vi "Gserver_main.vi"(8 "Database location":path=path "D:/Sgraph_database", 11 "DAQ-Queue":refnum<queue>) -> ()   [LabVIEW 2020, in "Gserver.lvclass"]
doc: "Gserver service.\n\nThis service will act on Gviewer queries.\nThis VI must be started to enable the Sgraph functionality\n\nUse the Close method of the Gserver class after the main application is ended to free all resources."
uses:
  Gserver.lvclass
  controls/Typedef_Gserver-init.ctl
  HISW/controls/typedef-DAQ-datagram.ctl
  HISW/controls/typedef-Qtype.ctl
  Gview/controls/Typedef_datarequest.ctl
  Gview/controls/Typedef_Live.ctl
  FAMM/controls/FAMM_reply_datagram.ctl
  FAMM/controls/FAMM_reply_WAQdata.ctl
  FAMM/controls/FAMM_reply_EAQdata.ctl
  FAMM/controls/FAMM_reply_PAQdata.ctl
  D:/Labview/Sgraph/Sgraph/source/Vsolver/Vsolver.lvclass
  Gserver.lvclass/Gserver.ctl
  Common/controls/MeMapInfo.ctl
  Common/controls/MMap_element.ctl
  FAMM/controls/typedef-functions.ctl
  controls/Typedef_Sgraph_Query.ctl
  Gview/controls/Typedef_Gserver-Replies.ctl
  Gview/controls/Typedef_ServerActions.ctl
  FAMM/FAMM.lvclass/FAMM.ctl
  FAMM/FAMM.lvclass
  HISW/HISW.lvclass
  FAMM/controls/typedef_FAMM_Query.ctl
  Common/controls/Global-services.vi
  Vsolver/Vsolver.lvclass
  Gview/Gviewer.lvclass
panel:
  out "Debug_Layer?":i32
  out "data 2":T1
  out "data":T6
  out "# elements in queue":i32
  out "Graphs Running":string[](array[string])
  out "Gserver":picture
  out "GserverInitState":T7
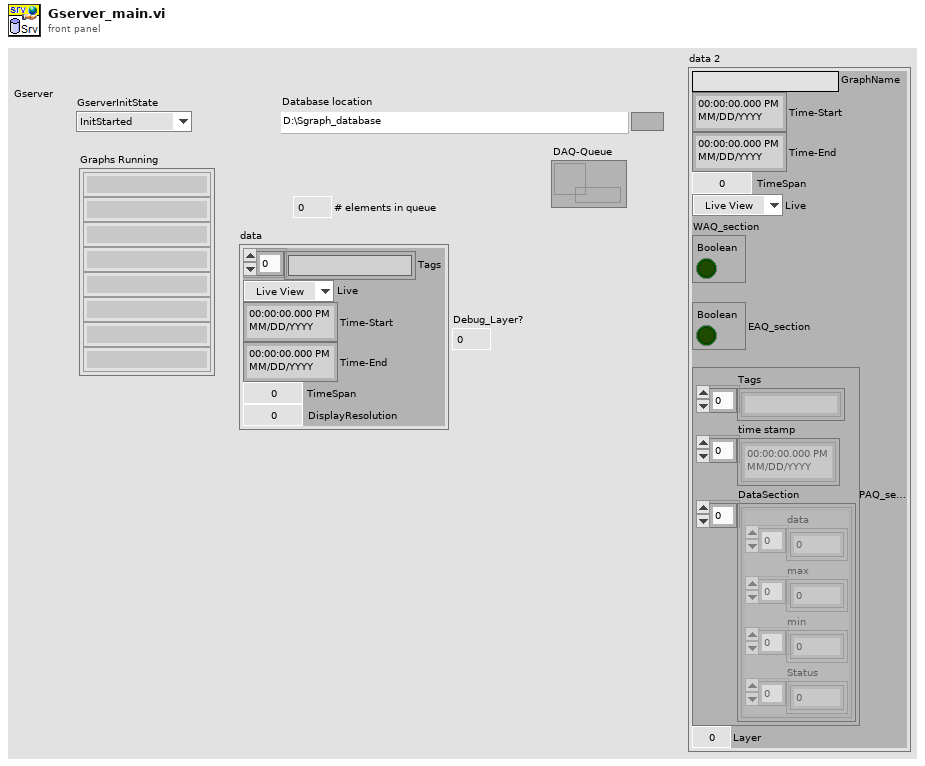
[diagram p1: front panel]
types:
  T1 = typedef "FAMM.lvclass/FAMM_reply_datagram.ctl" = cluster{"GraphName":string, "Time-Start":timestamp, "Time-End":timestamp, "TimeSpan":dbl, "Live":T2, "WAQ_section":T3, "EAQ_section":T4, "PAQ_section":T5, "Layer":i32}
  T2 = typedef "Gviewer.lvclass/Typedef_Live.ctl" = enum16{"Live View", "Freeze"}
  T3 = typedef "FAMM.lvclass/FAMM_reply_WAQdata.ctl" = cluster{"Boolean":bool}
  T4 = typedef "FAMM.lvclass/FAMM_reply_EAQdata.ctl" = cluster{"Boolean":bool}
  T5 = typedef "FAMM.lvclass/FAMM_reply_PAQdata.ctl" = cluster{"Tags":string[], "time stamp":timestamp[], "DataSection":cluster{"data":dbl[], "max":dbl[], "min":dbl[], "Status":u32[]}[]}
  T6 = typedef "Gviewer.lvclass/Typedef_datarequest.ctl" = cluster{"Tags":string[], "Live":T2, "Time-Start":timestamp, "Time-End":timestamp, "TimeSpan":dbl, "DisplayResolution":i32}
  T7 = typedef "Typedef_Gserver-init.ctl" = enum16{"InitStarted", "FAMM_started", "HISW_Started", "Active"}
  T8 = typedef "typedef-functions.ctl" = enum16{"PAQ-request", "PAQ-taglist-request", "WAQ-request", "EAQ-request", "TAG-based-request", "PAQ-MemoryMap", "Exit-FAMM"}
  T9 = typedef "MeMapInfo.ctl" = cluster{"MemLayer":T10[]}
  T10 = typedef "MMap_element.ctl" = cluster{"Name":string, "Length":i32, "Pointer":i32, "Tbegin":dbl, "Tend":dbl, "Tmin":dbl, "Tmax":dbl, "Tpnt-1":dbl, "Tpnt":dbl, "Tpnt+1":dbl}
  T11 = typedef "Gserver.lvclass/Typedef_Sgraph_Query.ctl" = cluster{"ViewportName":string, "Tags":string[], "Time-Start":timestamp, "Time-End":timestamp, "Pixels":i32, "Live":T2, "TimeSpan(sec)":dbl, "GViewer-Queue":refnum<queue>}
  T12 = typedef "Typedef_ServerActions.ctl" = enum16{"GraphUpdate", "SendAllTags", "SendIniPath", "SetGeneralOptions", "EditTagsOpen", "EditTagsPresetSave", "EditTagsPresetLoad", "EditTagsClose", "NewTagSelection", "ExitGraph"}
  T13 = typedef "Typedef_Gserver-Replies.ctl" = cluster{"ServerActions":T12, "data":variant, "Source":string, "Time Stamp":timestamp}
  T14 = typedef "typedef-Qtype.ctl" = enum16{"PAQ", "WAQ", "EAQ", "End-Service"}
  T15 = typedef "typedef-DAQ-datagram.ctl" = cluster{"Time Stamp":timestamp, "Source":string, "Data":variant, "Qtype":T14}
  T16 = typedef "typedef_FAMM_Query.ctl" = cluster{"Time Stamp":timestamp, "FAMM-function":T8, "Source":string, "Data":variant}
  T17 = typedef "Gserver.lvclass/Typedef_Gviewer-Query.ctl" = cluster{"Query_type":T18, "data":variant, "Source":string, "Time Stamp":timestamp}
  T18 = typedef "Gserver.lvclass/Typedef_QueryType.ctl" = enum16{"Subscribe", "DataRequest", "RequestAllTags", "RequestIniPath", "FAMMstarted", "SetClientOptions", "GviewerUpdate", "OpenNewGraph", "CloseClient", "CloseAllClients", "Close Gserver", "OpenMemoryMap", "MeMapDataRequest", "MeMapDataResponse"}
  T19 = typedef "FAMM.lvclass/Typedef_Gviewer_TagsUnits.ctl" = cluster{"PAQ_TAGs":string[], "WAQ_TAGs":string[], "EAQ_TAGs":string[], "PAQtagProps":T20[], "WAQtagProps":T20[], "EAQtagProps":T20[]}
  T20 = typedef "typedef_com_TagProp.ctl" = cluster{"Description":string, "EngUnits":string, "RangeH":dbl, "RangeL":dbl, "Resolution":i32, "Obsolete":bool, "ChangeDate":timestamp, "ChangeSource":string, "ChangeReason":string, "TagFunc":u32}
  T21 = cluster{"FAMM_PAQ_Layers":i32, "FAMM_PAQ_resolution":dbl}
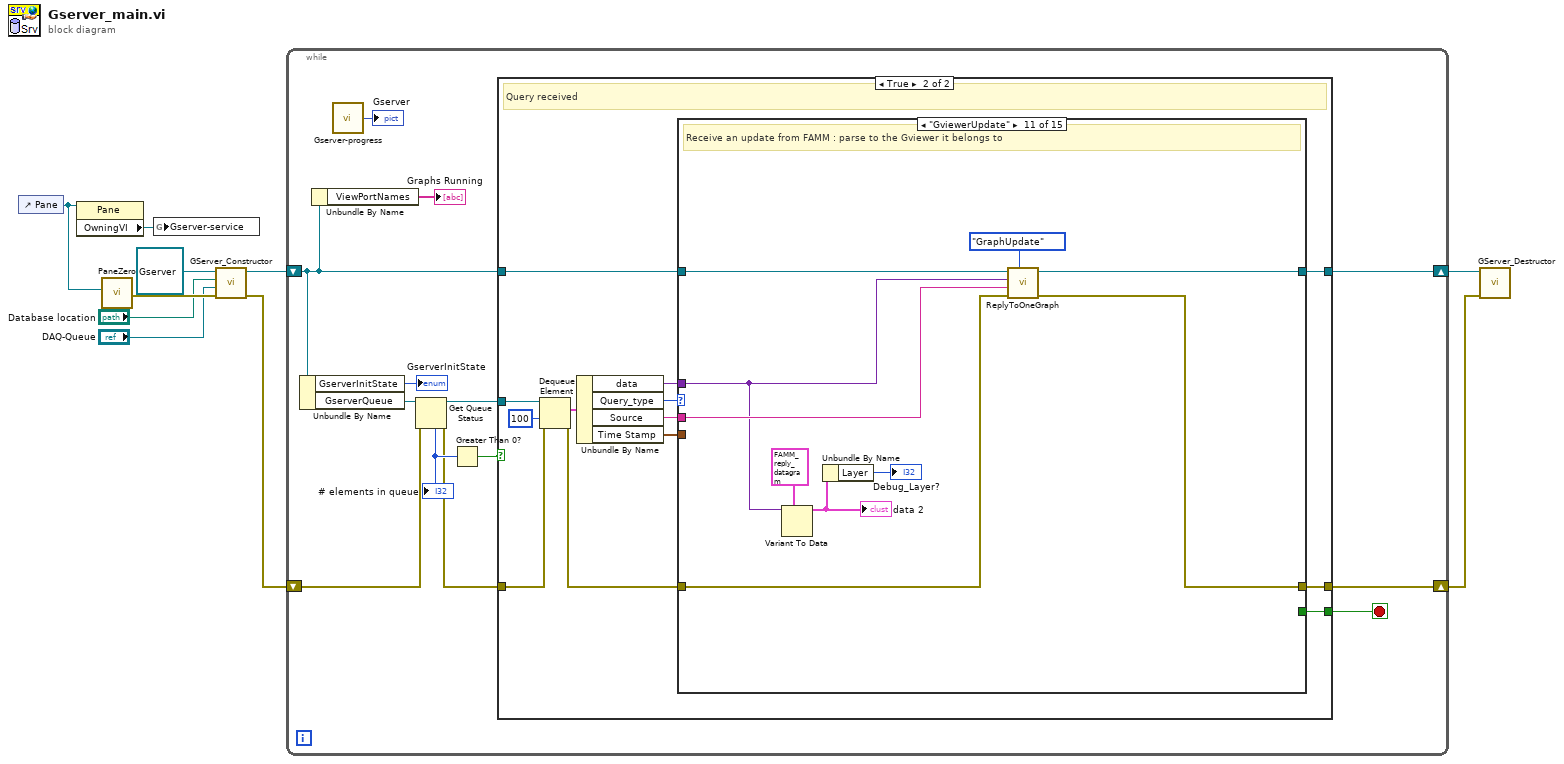
[diagram p0: block diagram]
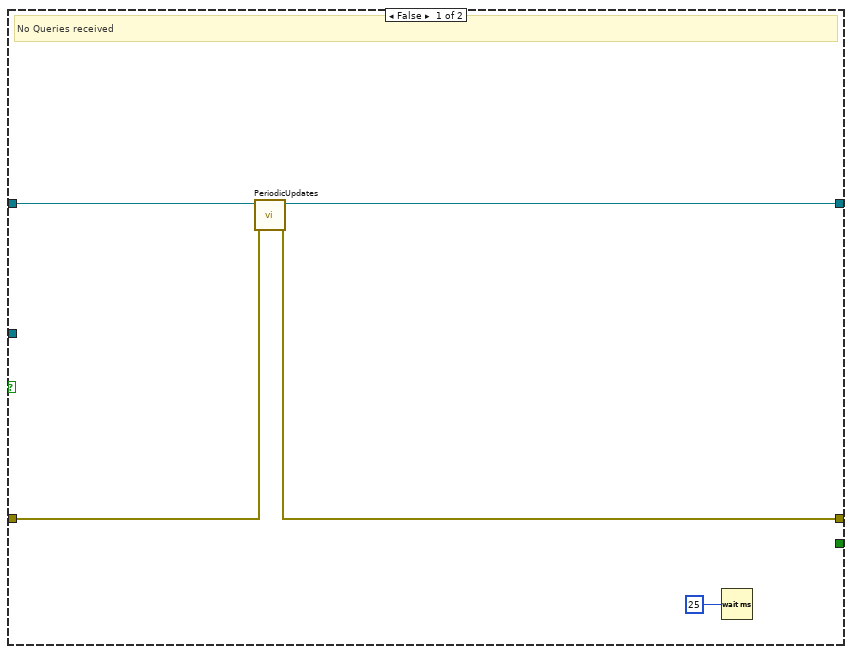
[diagram p2: hidden frame]
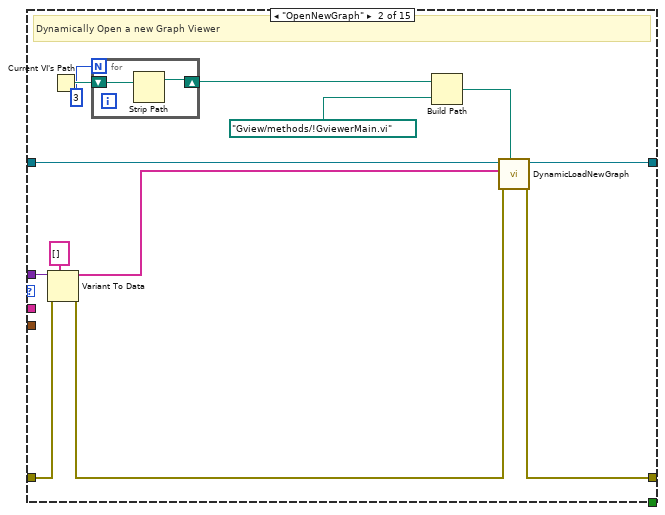
[diagram p4: hidden frame]
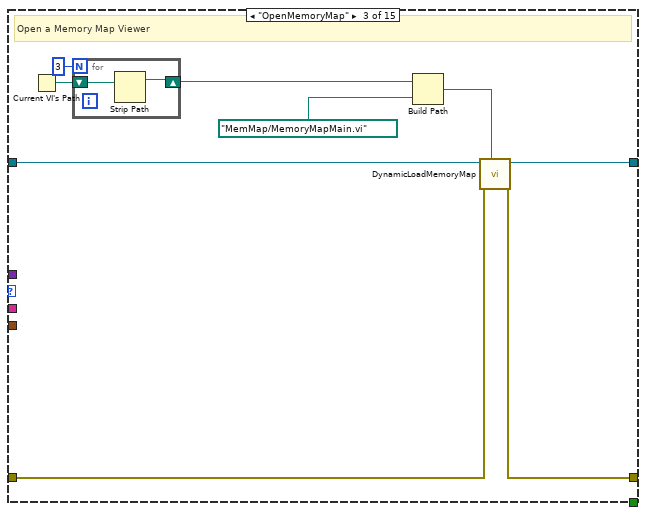
[diagram p5: hidden frame]
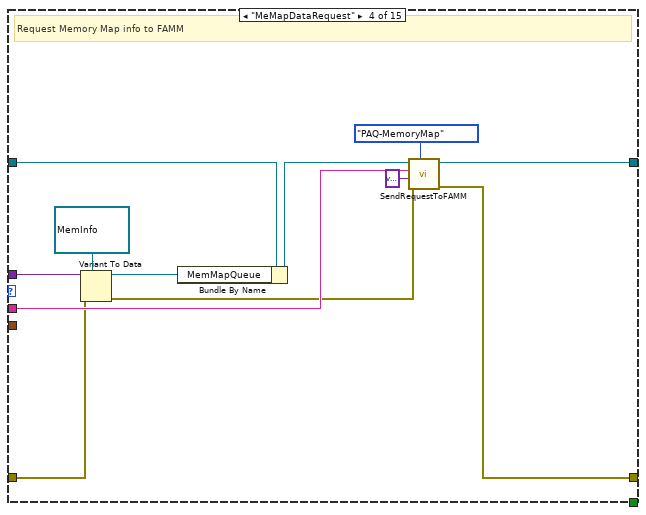
[diagram p6: hidden frame]
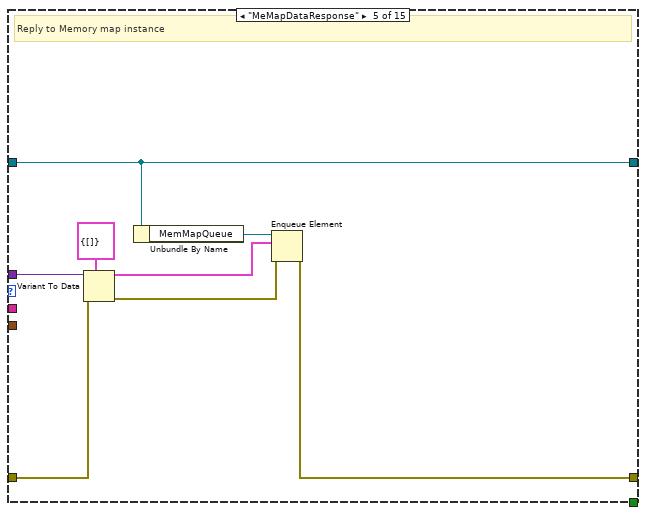
[diagram p7: hidden frame]
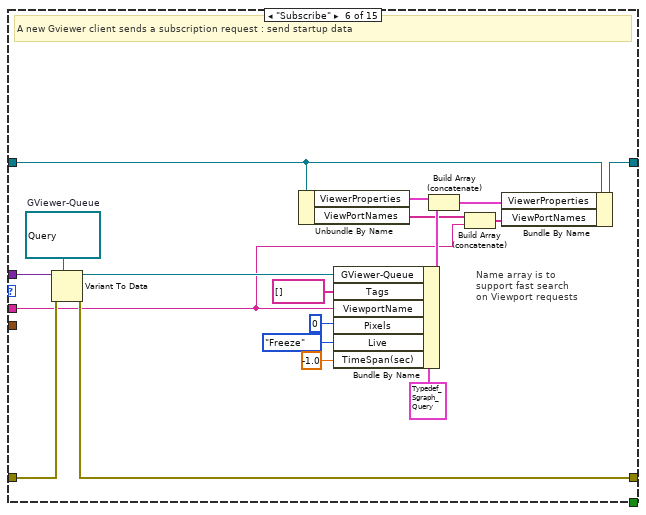
[diagram p8: hidden frame]
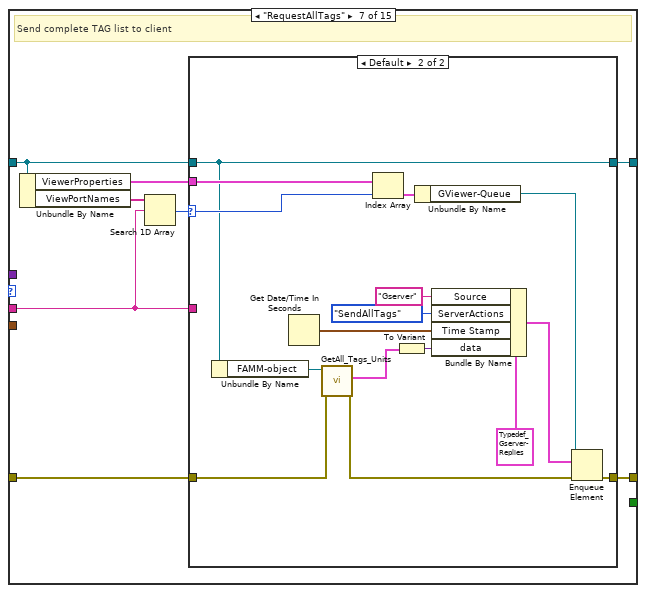
[diagram p9: hidden frame]
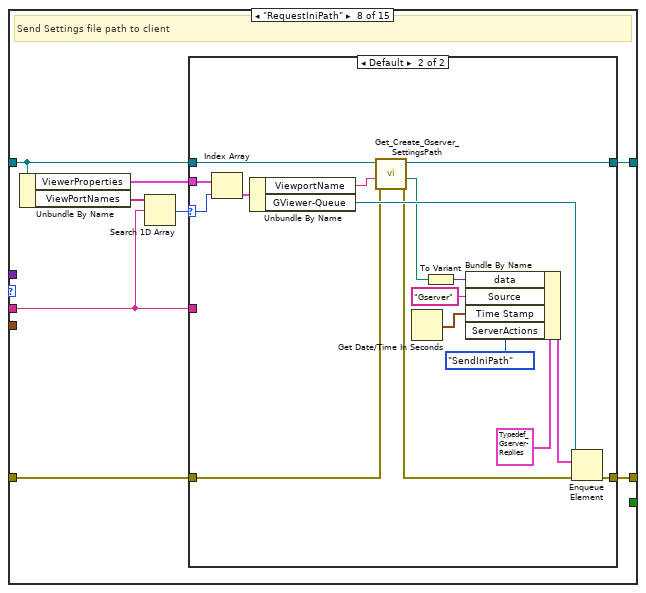
[diagram p11: hidden frame]
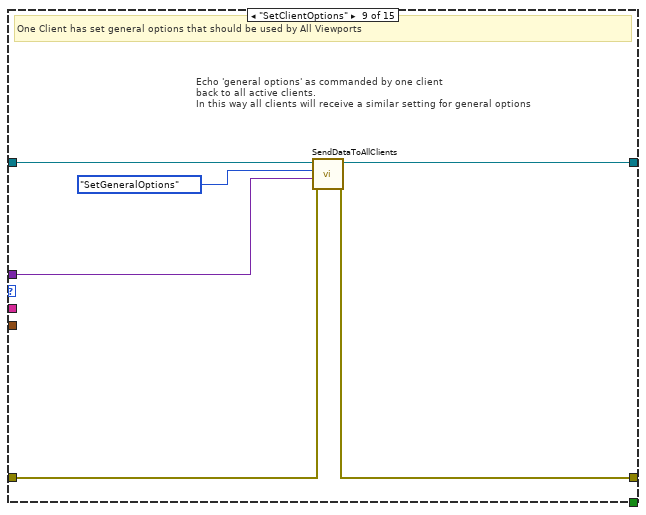
[diagram p13: hidden frame]
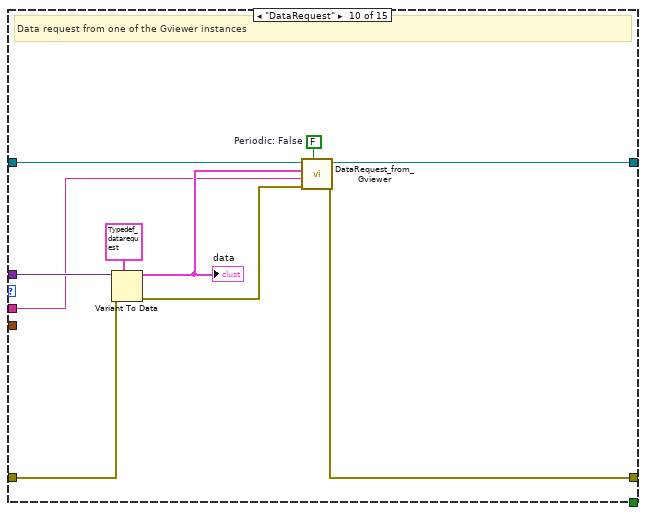
[diagram p14: hidden frame]
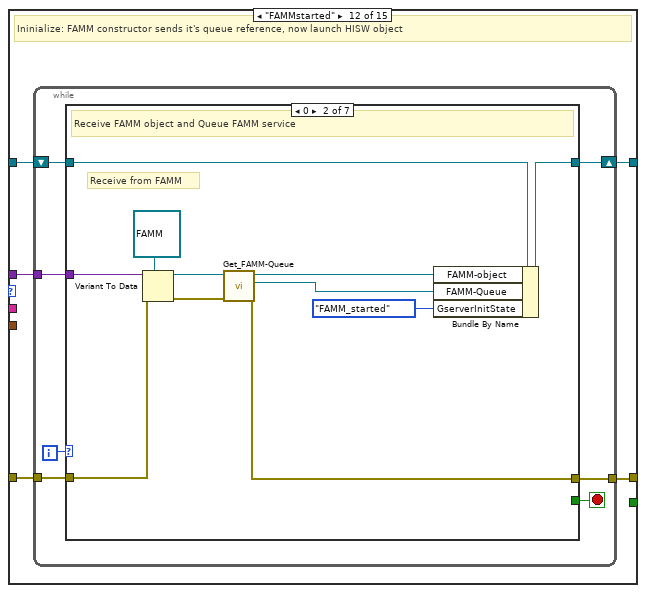
[diagram p15: hidden frame]
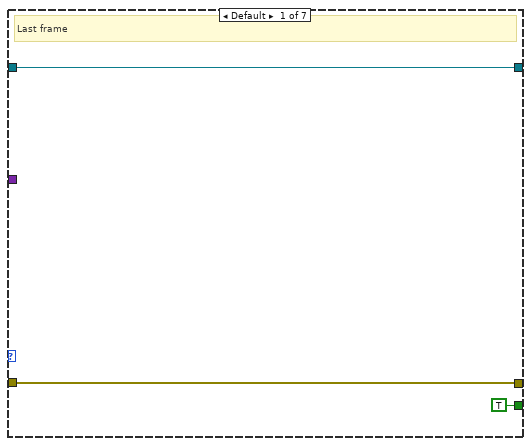
[diagram p16: hidden frame]
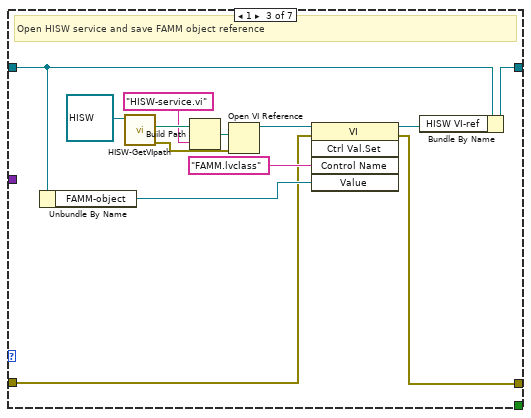
[diagram p17: hidden frame]
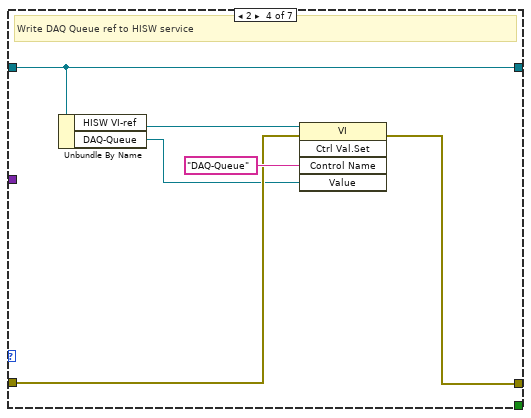
[diagram p18: hidden frame]
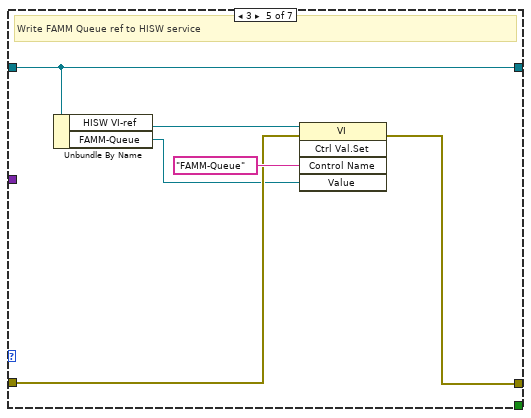
[diagram p19: hidden frame]
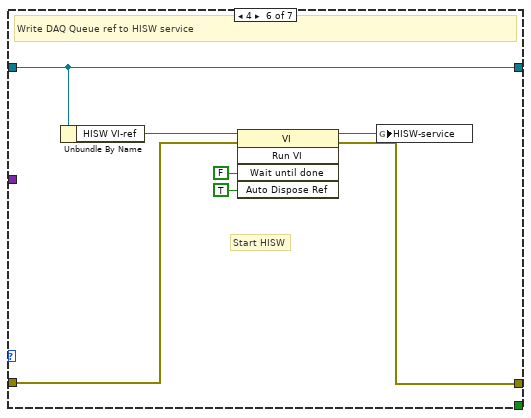
[diagram p20: hidden frame]
diagram:
  n1 = control-ref of="Pane"() -> (w3:refnum<vi>)
  n2 = property class="Pane"(reference=w3) -> ("OwningVI"=w5:refnum<vi>)  [unwired: 1 in, 2 out]
  n3 = call "PaneZero.vi"("Pane"=w3) -> ("error out"=w4:errorcluster)  [unwired: 10 in]
  n4 = global write "Global-services.vi" "Gserver-service"(w5) -> ()
  n5 = call "GServer_Constructor.vi"("error in (no error)"=w4, "DAQ-Queue"="DAQ-Queue", "Database location"="Database location", "Gserver in"=refnum<class "Gserver.lvclass"> refnum) -> ("error out"=w9:errorcluster, "Gserver out"=w10:refnum<class "Gserver.lvclass">)  [unwired: 6 in]
  n6 = while {
    shift-right: [w20] -> w8
    shift-left: w10 -> [w12]
    shift-right: [w19] -> w7
    shift-left: w9 -> [w17]
    stop <- w13 stop-if-true
    n7 = Unbundle By Name(w12) -> ("GserverInitState"=→"GserverInitState":T7, "GserverQueue"=w23:refnum<queue>)
    n8 = Unbundle By Name(w12) -> ("ViewPortNames"=→"Graphs Running":string[])
    n9 = call "Gserver-progress.vi"() -> ("37x37"=→"Gserver":picture)  [unwired: 7 in]
    n10 = Get Queue Status(queue=w23, error in (no error)=w17) -> (queue out=w18:refnum<queue>, error out=w16:errorcluster, # elements in queue=w22:i32)  [unwired: 1 in, 5 out]
    "# elements in queue" <- w22
    n11 = Greater Than 0?(x=w22) -> (x > 0?=w21:bool)
    n12 = case shown="True" w21 {
      tunnel: w12 -> [w27 w35]
      tunnel: w16 -> [w26 w39]
      tunnel: [w25 w33] -> w20
      tunnel: [w24 w34] -> w19
      tunnel: w18 -> [_ w41]
      tunnel: [_ w30] -> w13
      frame False {
        # "No Queries received"
        n13 = call "PeriodicUpdates.vi"("error in (no error)"=w26, "Gserver in"=w27) -> ("error out"=w24:errorcluster, "Gserver out"=w25:refnum<class "Gserver.lvclass">)  [unwired: 8 in]
        n14 = Wait (ms)(milliseconds to wait=u32 25) -> ()  [unwired: 1 out]
      }
      frame True {
        # "Query received"
        n15 = Dequeue Element(queue=w41, timeout in ms (-1)=100, error in (no error)=w39) -> (element=w38:T17, error out=w36:errorcluster)  [unwired: 2 out]
        n16 = Unbundle By Name(w38) -> ("data"=w32:variant, "Query_type"=w37:T18, "Source"=w29:string, "Time Stamp"=w31:timestamp)
        n17 = case shown="\"GviewerUpdate\"" w37 {
          tunnel: w36 -> [w42 w44 w60 w71 w82 w93 w111 w137 w162 w174 w182 w188 w255 w261 w272]
          tunnel: w35 -> [w43 w49 w62 w78 w89 w107 w113 w139 w166 w172 w186 w190 w257 w260 w271]
          tunnel: [w42 w48 w61 w72 w83 w94 w110 w136 w161 w168 w184 w187 w254 w258 w269] -> w34
          tunnel: [w43 w50 w63 w75 w89 w106 w112 w138 w165 w173 w185 w191 w256 w259 w270] -> w33
          tunnel: w32 -> [_ w56 _ w81 w87 w97 _ _ w163 w176 w179 w189 _ _ _]
          tunnel: w31 -> [_ _ _ _ _ _ _ _ _ _ _ _ _ _ _]
          tunnel: [_ _ _ _ _ _ _ _ _ _ _ _ _ _ w268] -> w30
          tunnel: w29 -> [_ _ _ w74 _ w90 w114 w140 _ w169 w183 _ w253 _ _]
          frame Default {
            # "Not implemented"
          }
          frame "OpenNewGraph" {
            # "Dynamically Open a new Graph Viewer"
            n18 = Variant To Data(error in=w44, type=string[] [], Variant=w56) -> (data=w46:string[], error out=w45:errorcluster)
            n19 = Current VI's Path() -> (path=w54:path)
            n20 = for {
              N: 3 -> [_]
              shift-right: [w57] -> w52
              shift-left: w54 -> [w58]
              n21 = Strip Path(path=w58) -> (stripped path=w57:path)  [unwired: 1 out]
            }
            n22 = Build Path(base path=w52, name or relative path=path "Gview/methods/!GviewerMain.vi") -> (appended path=w47:path)
            n23 = call "DynamicLoadNewGraph.vi"("ViewerPath"=w47, "error in (no error)"=w45, "Preferred_tags"=w46, "Gserver in"=w49) -> ("error out"=w48:errorcluster, "Gserver out"=w50:refnum<class "Gserver.lvclass">)  [unwired: 6 in]
          }
          frame "OpenMemoryMap" {
            # "Open a Memory Map Viewer"
            n24 = Current VI's Path() -> (path=w67:path)
            n25 = for {
              N: 3 -> [_]
              shift-right: [w68] -> w65
              shift-left: w67 -> [w69]
              n26 = Strip Path(path=w69) -> (stripped path=w68:path)  [unwired: 1 out]
            }
            n27 = Build Path(base path=w65, name or relative path=path "MemMap/MemoryMapMain.vi") -> (appended path=w59:path)
            n28 = call "DynamicLoadMemoryMap.vi"("ApplicationPath"=w59, "error in (no error)"=w60, "Gserver in"=w62) -> ("error out"=w61:errorcluster, "Gserver out"=w63:refnum<class "Gserver.lvclass">)  [unwired: 7 in]
          }
          frame "MeMapDataRequest" {
            # "Request Memory Map info to FAMM"
            n29 = Variant To Data(error in=w71, type=refnum<queue> refnum ("queue out"), Variant=w81) -> (data=w79:refnum<queue>, error out=w73:errorcluster)
            n30 = Bundle By Name(cluster=w78, "MemMapQueue"=w79) -> (w76:refnum<class "Gserver.lvclass">)
            n31 = call "SendRequestToFAMM.vi"("FAMM-function"=typedef-functions."PAQ-MemoryMap", "error in (no error)"=w73, "Data"=variant, "Source"=w74, "Gserver in"=w76) -> ("error out"=w72:errorcluster, "Gserver out"=w75:refnum<class "Gserver.lvclass">)  [unwired: 5 in]
          }
          frame "MeMapDataResponse" {
            # "Reply to Memory map instance"
            n32 = Variant To Data(error in=w82, type=T9 {"MemLayer"=[]} ("element"), Variant=w87) -> (data=w84:T9, error out=w85:errorcluster)
            n33 = Unbundle By Name(w89) -> ("MemMapQueue"=w88:refnum<queue>)
            n34 = Enqueue Element(queue=w88, element=w84, error in (no error)=w85) -> (error out=w83:errorcluster)  [unwired: 1 in, 2 out]
          }
          frame "Subscribe" {
            w98 = refnum<queue> refnum  # GViewer-Queue
            # "Name array is to\nsupport fast search\non Viewport requests"
            # "A new Gviewer client sends a subscription request : send startup data"
            n35 = Variant To Data(error in=w93, type=w98, Variant=w97) -> (data=w96:refnum<queue>, error out=w94:errorcluster)
            n36 = Unbundle By Name(w107) -> ("ViewerProperties"=w105:T11[], "ViewPortNames"=w92:string[])
            n37 = Bundle By Name(cluster=T11 {"ViewportName"="", "Tags"=[], "Time-Start"=timestamp(0 s since 1904-01-01), "Time-End"=timestamp(0 s since 1904-01-01), "Pixels"=0, "Live"=enum."Live View", "TimeSpan(sec)"=0.0, "GViewer-Queue"=refnum} ("Query_datagram"), "GViewer-Queue"=w96, "Tags"=string[] [], "ViewportName"=w90, "Pixels"=0, "Live"=Typedef_Live."Freeze", "TimeSpan(sec)"=-1.0) -> (w102:T11)
            n38 = Build Array (concatenate)(w105, w102) -> (w104:T11[])
            n39 = Build Array (concatenate)(w92, w90) -> (w91:string[])
            n40 = Bundle By Name(cluster=w107, "ViewerProperties"=w104, "ViewPortNames"=w91) -> (w106:refnum<class "Gserver.lvclass">)
          }
          frame "RequestAllTags" {
            # "Send complete TAG list to client"
            n41 = Unbundle By Name(w113) -> ("ViewerProperties"=w109:T11[], "ViewPortNames"=w115:string[])
            n42 = Search 1D Array(1D array=w115, element=w114) -> (index of element=w108:i32)  [unwired: 1 in]
            n43 = case shown="Default" w108 {
              selector: w108 -> [_ w132]
              tunnel: w114 -> [_ _]
              tunnel: w113 -> [w117 w128]
              tunnel: [w117 w128] -> w112
              tunnel: w111 -> [w116 w120]
              tunnel: [w116 w129] -> w110
              tunnel: w109 -> [_ w133]
              frame -1 {
              }
              frame Default {
                n44 = Unbundle By Name(w128) -> ("FAMM-object"=w121:refnum<class "FAMM.lvclass">)
                n45 = Get Date/Time In Seconds() -> (seconds since 1Jan1904=w124:timestamp)
                n46 = call "GetAll_Tags_Units.vi"("error in (no error)"=w120, "FAMM in"=w121) -> ("error out"=w119:errorcluster, "Tags_Units"=w118:T19)  [unwired: 7 in, 1 out]
                n47 = Index Array(array=w133, index=w132) -> (element=w131:T11)
                n48 = To Variant(anything=w118) -> (Variant=w122:variant)
                n49 = Unbundle By Name(w131) -> ("GViewer-Queue"=w130:refnum<queue>)
                n50 = Bundle By Name(cluster=T13 {"ServerActions"=enum."GraphUpdate", "data"=variant, "Source"="", "Time Stamp"=timestamp(0 s since 1904-01-01)} ("element"), "Source"="Gserver", "ServerActions"=Typedef_ServerActions."SendAllTags", "Time Stamp"=w124, "data"=w122) -> (w126:T13)
                n51 = Enqueue Element(queue=w130, element=w126, error in (no error)=w119) -> (error out=w129:errorcluster)  [unwired: 1 in, 2 out]
              }
            }
          }
          frame "RequestIniPath" {
            # "Send Settings file path to client"
            n52 = Unbundle By Name(w139) -> ("ViewerProperties"=w135:T11[], "ViewPortNames"=w141:string[])
            n53 = Search 1D Array(1D array=w141, element=w140) -> (index of element=w134:i32)  [unwired: 1 in]
            n54 = case shown="Default" w134 {
              selector: w134 -> [_ w159]
              tunnel: w140 -> [_ _]
              tunnel: w139 -> [w143 w151]
              tunnel: [w143 w152] -> w138
              tunnel: w137 -> [w142 w148]
              tunnel: [w142 w156] -> w136
              tunnel: w135 -> [_ w160]
              frame -1 {
              }
              frame Default {
                n55 = Index Array(array=w160, index=w159) -> (element=w158:T11)
                n56 = Unbundle By Name(w158) -> ("ViewportName"=w150:string, "GViewer-Queue"=w157:refnum<queue>)
                n57 = call "Get_Create_Gserver_SettingsPath.vi"("error in (no error)"=w148, "ViewPortName"=w150, "Gserver in"=w151) -> ("error out"=w149:errorcluster, "Viewport settings path"=w144:path, "Gserver out"=w152:refnum<class "Gserver.lvclass">)  [unwired: 6 in]
                n58 = Get Date/Time In Seconds() -> (seconds since 1Jan1904=w146:timestamp)
                n59 = To Variant(anything=w144) -> (Variant=w147:variant)
                n60 = Bundle By Name(cluster=T13 {"ServerActions"=enum."GraphUpdate", "data"=variant, "Source"="", "Time Stamp"=timestamp(0 s since 1904-01-01)} ("element"), "data"=w147, "Source"="Gserver", "Time Stamp"=w146, "ServerActions"=Typedef_ServerActions."SendIniPath") -> (w154:T13)
                n61 = Enqueue Element(queue=w157, element=w154, error in (no error)=w149) -> (error out=w156:errorcluster)  [unwired: 1 in, 2 out]
              }
            }
          }
          frame "SetClientOptions" {
            # "Echo 'general options' as commanded by one client\nback to all active clients.\nIn this way all clients will receive a similar setting for general options"
            # "One Client has set general options that should be used by All Viewports"
            n62 = call "SendDataToAllClients.vi"("error in (no error)"=w162, "data"=w163, "ServerActions"=Typedef_ServerActions."SetGeneralOptions", "Gserver in"=w166) -> ("error out"=w161:errorcluster, "Gserver out"=w165:refnum<class "Gserver.lvclass">)  [unwired: 6 in]
          }
          frame "DataRequest" {
            w167 = FALSE  # Periodic: False
            # "Data request from one of the Gviewer instances"
            n63 = Variant To Data(error in=w174, type=T6 {"Tags"=[], "Live"=enum."Live View", "Time-Start"=timestamp(0 s since 1904-01-01), "Time-End"=timestamp(0 s since 1904-01-01), "TimeSpan"=0.0, "DisplayResolution"=0} ("Cluster"), Variant=w176) -> (data=w171:T6, error out=w170:errorcluster)
            "data" <- w171
            n64 = call "DataRequest_from_Gviewer.vi"("Periodic?"=w167, "error in (no error)"=w170, "Sending Gviewer"=w169, "DataRequest"=w171, "Gserver in"=w172) -> ("error out"=w168:errorcluster, "Gserver out"=w173:refnum<class "Gserver.lvclass">)  [unwired: 5 in]
          }
          frame "GviewerUpdate" {
            # "Receive an update from FAMM : parse to the Gviewer it belongs to"
            n65 = Variant To Data(type=T1 {"GraphName"="", "Time-Start"=timestamp(0 s since 1904-01-01), "Time-End"=timestamp(0 s since 1904-01-01), "TimeSpan"=0.0, "Live"=enum."Live View", "WAQ_section"={"Boolean"=FALSE}, "EAQ_section"={"Boolean"=FALSE}, "PAQ_section"={"Tags"=[], "time stamp"=[], "DataSection"=[]}, "Layer"=0} ("GviewerUpdate"), Variant=w179) -> (data=w178:T1)  [unwired: 1 in, 1 out]
            "data 2" <- w178
            n66 = Unbundle By Name(w178) -> ("Layer"=→"Debug_Layer?":i32)
            n67 = call "ReplyToOneGraph.vi"("ServerActions"=Typedef_ServerActions."GraphUpdate", "error in (no error)"=w182, "Graph name"=w183, "data"=w179, "Gserver in"=w186) -> ("error out"=w184:errorcluster, "Gserver out"=w185:refnum<class "Gserver.lvclass">)  [unwired: 5 in]
          }
          frame "FAMMstarted" {
            # "Ininialize: FAMM constructor sends it's queue reference, now launch HISW object"
            n68 = while {
              tunnel: w189 -> [w196]
              tunnel: w188 -> [w195]
              shift-right: [w198] -> w191
              shift-left: w190 -> [w197]
              tunnel: [w192] -> w187
              i -> [w194]
              stop <- w193 stop-if-true
              n69 = case shown="0" w194 {
                tunnel: [w201 w212 w215 w229 w235 w244 w246] -> w198
                tunnel: w197 -> [w201 w210 w214 w229 w235 w244 w245]
                tunnel: w196 -> [_ w209 _ _ _ _ _]
                tunnel: w195 -> [w199 w208 w217 w230 w236 w240 w250]
                tunnel: [TRUE _ _ _ _ _ _] -> w193
                tunnel: [w199 w204 w213 w226 w232 w239 w251] -> w192
                frame Default {
                  # "Last frame"
                }
                frame 0 {
                  # "Receive from FAMM"
                  # "Receive FAMM object and Queue FAMM service"
                  n70 = Variant To Data(error in=w208, type=refnum<class "FAMM.lvclass"> refnum ("FAMM out"), Variant=w209) -> (data=w206:refnum<class "FAMM.lvclass">, error out=w205:errorcluster)
                  n71 = call-dynamic "Get_FAMM-Queue.vi"("error in (no error)"=w205, "FAMM in"=w206) -> ("error out"=w204:errorcluster, "FAMM-Queue"=w202:refnum<queue>, "FAMM out"=w203:refnum<class "FAMM.lvclass">)  [unwired: 7 in]
                  n72 = Bundle By Name(cluster=w210, "FAMM-object"=w203, "FAMM-Queue"=w202, "GserverInitState"=Typedef_Gserver-init."FAMM_started") -> (w212:refnum<class "Gserver.lvclass">)
                }
                frame 1 {
                  # "Open HISW service and save FAMM object reference"
                  n73 = Unbundle By Name(w214) -> ("FAMM-object"=w218:refnum<class "FAMM.lvclass">)
                  n74 = call "HISW-GetVIpath.vi"("HISW in"=refnum<class "HISW.lvclass"> refnum) -> ("error out"=w223:errorcluster, "MethodsPath"=w224:path)  [unwired: 8 in, 1 out]
                  n75 = Build Path(base path=w224, name or relative path="HISW-service.vi") -> (appended path=w225:path)
                  n76 = Open VI Reference(vi path=w225, error in (no error)=w223) -> (vi reference=w222:refnum<vi>)  [unwired: 4 in, 1 out]
                  n77 = invoke class="VI" method="Ctrl Val.Set"(reference=w222, error in=w217, "Control Name"="FAMM.lvclass", "Value"=w218) -> (reference out=w216:refnum<vi>, error out=w213:errorcluster)  [unwired: 1 in, 3 out]
                  n78 = Bundle By Name(cluster=w214, "HISW VI-ref"=w216) -> (w215:refnum<class "Gserver.lvclass">)
                }
                frame 2 {
                  # "Write DAQ Queue ref to HISW service"
                  n79 = Unbundle By Name(w229) -> ("HISW VI-ref"=w228:refnum<vi>, "DAQ-Queue"=w227:refnum<queue>)
                  n80 = invoke class="VI" method="Ctrl Val.Set"(reference=w228, error in=w230, "Control Name"="DAQ-Queue", "Value"=w227) -> (error out=w226:errorcluster)  [unwired: 1 in, 4 out]
                }
                frame 3 {
                  # "Write FAMM Queue ref to HISW service"
                  n81 = Unbundle By Name(w235) -> ("HISW VI-ref"=w234:refnum<vi>, "FAMM-Queue"=w233:refnum<queue>)
                  n82 = invoke class="VI" method="Ctrl Val.Set"(reference=w234, error in=w236, "Control Name"="FAMM-Queue", "Value"=w233) -> (error out=w232:errorcluster)  [unwired: 1 in, 4 out]
                }
                frame 4 {
                  # "Start HISW"
                  # "Write DAQ Queue ref to HISW service"
                  n83 = Unbundle By Name(w244) -> ("HISW VI-ref"=w241:refnum<vi>)
                  n84 = invoke class="VI" method="Run VI"(reference=w241, error in=w240, "Wait until done"=FALSE ("Wait Until Done"), "Auto Dispose Ref"=TRUE ("Auto Dispose Reference")) -> (reference out=w238:refnum<vi>, error out=w239:errorcluster)  [unwired: 1 in, 3 out]
                  n85 = global write "Global-services.vi" "HISW-service"(w238) -> ()
                }
                frame 5 {
                  # "Get FAMM PAQ resolution data"
                  n86 = Unbundle By Name(w245) -> ("FAMM-object"=w252:refnum<class "FAMM.lvclass">)
                  n87 = call "GetPAQresolution.vi"("error in (no error)"=w250, "FAMM in"=w252) -> ("error out"=w251:errorcluster, "PAQ-resolution"=w249:T21)  [unwired: 7 in, 1 out]
                  n88 = Unbundle By Name(w249) -> ("FAMM_PAQ_Layers"=w248:i32, "FAMM_PAQ_resolution"=w247:dbl)
                  n89 = Bundle By Name(cluster=w245, "FAMM_PAQ_Layers"=w248, "FAMM_PAQ_resolution"=w247) -> (w246:refnum<class "Gserver.lvclass">)
                }
              }
            }
          }
          frame "CloseClient" {
            # "Graph display request to close the graph"
            n90 = call "CloseOneGraph.vi"("error in (no error)"=w255, "Graph name"=w253, "Gserver in"=w257) -> ("error out"=w254:errorcluster, "Gserver out"=w256:refnum<class "Gserver.lvclass">)  [unwired: 7 in]
          }
          frame "CloseAllClients" {
            # "One Graph display requests to close all Graphs"
            n91 = Unbundle By Name(w260) -> ("ViewPortNames"=w262:string[])
            n92 = for "Loop over all viewports and perform a clean Graph Close" {
              tunnel: w262 -> [w266] mode=indexing
              shift-right: [w263] -> w259
              shift-left: w260 -> [w267]
              shift-right: [w264] -> w258
              shift-left: w261 -> [w265]
              n93 = call "CloseOneGraph.vi"("error in (no error)"=w265, "Graph name"=w266, "Gserver in"=w267) -> ("error out"=w264:errorcluster, "Gserver out"=w263:refnum<class "Gserver.lvclass">)  [unwired: 7 in]
            }
          }
          frame "Close Gserver" {
            # "Close the SGraph server"
            n94 = while {
              shift-right: [w276] -> w269
              shift-left: w272 -> [w277]
              shift-right: [w274] -> w270
              shift-left: w271 -> [w275]
              tunnel: [w273] -> w268
              i -> [w278]
              stop <- w273 stop-if-true
              n95 = case shown="2" w278 {
                tunnel: [TRUE _ _ _] -> w273
                tunnel: w277 -> [w280 w291 w299 w302]
                tunnel: [w280 w289 w298 w303] -> w276
                tunnel: w275 -> [w279 w292 w301 w305]
                tunnel: [w279 w283 w301 w306] -> w274
                frame Default {
                  # "Last frame: no code here"
                }
                frame 0 {
                  # "Close Vsolver class, End HISW service"
                  n96 = call "Vsolver_destructor.vi"("error in (no error)"=w291, "Vsolver in"=w292) -> ("error out"=w290:errorcluster, "Vsolver out"=w283:refnum<class "Gserver.lvclass">)  [unwired: 8 in]
                  n97 = Get Date/Time In Seconds() -> (seconds since 1Jan1904=w287:timestamp)
                  n98 = Unbundle By Name(w283) -> ("DAQ-Queue"=w282:refnum<queue>)
                  n99 = Bundle By Name(cluster=T15 {"Time Stamp"=timestamp(0 s since 1904-01-01), "Source"="", "Data"=variant, "Qtype"=enum."PAQ"} ("element"), "Time Stamp"=w287, "Source"="Gserver", "Qtype"=typedef-Qtype."End-Service") -> (w284:T15)
                  n100 = Enqueue Element(queue=w282, element=w284, error in (no error)=w290) -> (error out=w289:errorcluster)  [unwired: 1 in, 2 out]
                }
                frame 1 {
                  # "Exit FAMM service"
                  n101 = Get Date/Time In Seconds() -> (seconds since 1Jan1904=w296:timestamp)
                  n102 = Bundle By Name(cluster=T16 {"Time Stamp"=timestamp(0 s since 1904-01-01), "FAMM-function"=enum."PAQ-request", "Source"="", "Data"=variant} ("element"), "FAMM-function"=typedef-functions."Exit-FAMM", "Source"="Gserver", "Time Stamp"=w296) -> (w293:T16)
                  n103 = Unbundle By Name(w301) -> ("FAMM-Queue"=w300:refnum<queue>)
                  n104 = Enqueue Element(queue=w300, element=w293, error in (no error)=w299) -> (error out=w298:errorcluster)  [unwired: 1 in, 2 out]
                }
                frame 2 {
                  # "Exit Viewport Applications"
                  n105 = call "SendDataToAllClients.vi"("error in (no error)"=w302, "ServerActions"=Typedef_ServerActions."ExitGraph", "Gserver in"=w305) -> ("error out"=w303:errorcluster, "Gserver out"=w306:refnum<class "Gserver.lvclass">)  [unwired: 7 in]
                }
              }
            }
          }
        }
      }
    }
  }
  n106 = call "GServer_Destructor.vi"("error in (no error)"=w7, "Gserver in"=w8) -> ()  [unwired: 8 in, 2 out]
